vi "Send Data.vi"(7 "Data DVR":refnum<data-value>, 8 "Error In":errorcluster, 11 "Stream Data in":refnum<class "Stream Data.lvclass">) -> (0 "Error Out":errorcluster, 3 "Stream Data out":refnum<class "Stream Data.lvclass">)   [LabVIEW 2020, in "Stream Data.lvclass"]
doc: "The method streams data to the receiver class"
uses:
  Stream Data.lvclass
  Controls/Queue Operation.ctl
  Data/Data.lvclass
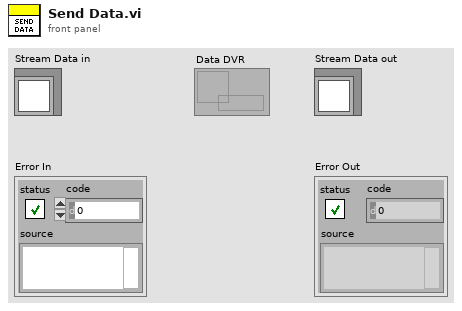
[diagram p1: front panel]
types:
  T1 = typedef "Queue Operation.ctl" = enum16{"Create & Enqueue N", "Enqueue N", "Dequeue", "Enstack N", "Flush", "Release"}
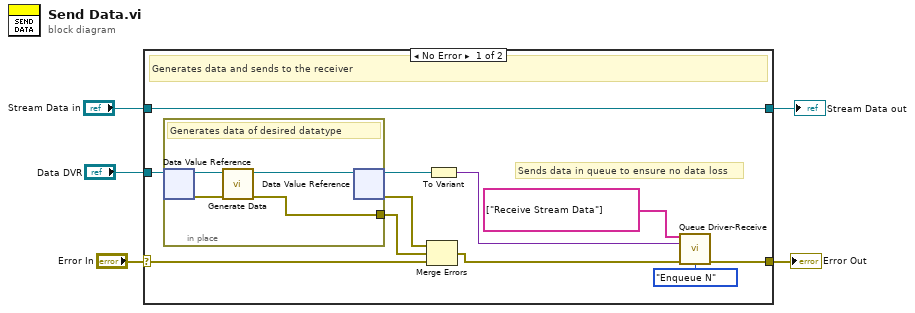
[diagram p0: block diagram]
diagram:
  n1 = case shown="No Error" "Error In" {
    selector: "Error In" -> [w16 w22]
    tunnel: [w10 w22] -> w4
    tunnel: [w15 w21] -> w2
    tunnel: "Stream Data in" -> [w15 w21]
    tunnel: "Data DVR" -> [w14 _]
    frame No Error {
      # "Sends data in queue to ensure no data loss"
      # "Generates data and sends to the receiver"
      n2 = in-place {
        in-place-border: [w20] -> w11
        # "Generates data of desired datatype"
        n3 = in-place-dvr #1(w14) -> (w18:refnum<class "Data.lvclass">, w19:errorcluster)
        n4 = call-dynamic "Generate Data.vi"("Error In"=w19, "Data in"=w18) -> ("Error Out"=w20:errorcluster, "Data out"=w17:refnum<class "Data.lvclass">)  [unwired: 8 in]
        n5 = in-place-dvr #1(w17) -> (w9:refnum<data-value>, w12:errorcluster)
      }
      n6 = Merge Errors(w12, w11, w16) -> (w13:errorcluster)
      n7 = To Variant(anything=w9) -> (Variant=w8:variant)
      n8 = call "Queue Driver-Receive.vi"("States[]"=string[] ["Receive Stream Data"], "Data"=w8, "Error In"=w13, "Queue Operation"=Queue_Operation."Enqueue N") -> ("Error Out"=w10:errorcluster)  [unwired: 10 in, 1 out]
    }
    frame Error {
    }
  }
  "Error Out" <- w4
  "Stream Data out" <- w2
